vi "ODE Solver main.vi"(5 "data":variant, 7 "ODE F(X,t)":refnum<vi>, 8 "error in (no error)":errorcluster, 10 "simulation parameters":T1={"Initial Time"=0.0, "Final Time"=10.0, "Time Step"=0.1, "Absolute Tolerance"=0.001, "Relative Tolerance"=0.001, "Continuous Solver"=enum."Runge-Kutta 45 (variable)", "Discrete Time Step"=1.0, "Minimum Time Step"=1e-08, "Maximum Time Step"=1.0, "Initial Time Step"=0.01} {"Initial Time Step" min=0.0; "Maximum Time Step" min=0.0}, 11 "x0":dbl[](array[numeric])) -> (0 "error out":errorcluster, 2 "outputs":dbl[][](array[numeric]), 3 "times":dbl[](array[numeric]))   [LabVIEW 2010, in "NI_Gmath.lvlib"]
doc: "Solves ordinary differential equations with initial conditions of the following form: X'=F(X,t). You must manually select the polymorphic instance to use."
uses:
  NI_Gmath.lvlib
  SIM Diagram Parameters.ctl
  SIM Continuous Solvers.ctl
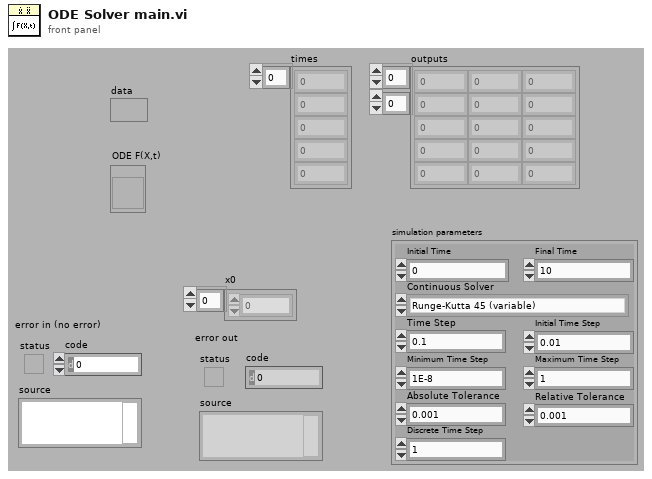
[diagram p1: front panel]
types:
  T1 = typedef "SIM Diagram Parameters.ctl" = cluster{"Initial Time":dbl, "Final Time":dbl, "Time Step":dbl, "Absolute Tolerance":dbl, "Relative Tolerance":dbl, "Continuous Solver":T2, "Discrete Time Step":dbl, "Minimum Time Step":dbl, "Maximum Time Step":dbl, "Initial Time Step":dbl}
  T2 = typedef "SIM Continuous Solvers.ctl" = enum16{"Runge-Kutta 1 (Euler)", "Runge-Kutta 2", "Runge-Kutta 3", "Runge-Kutta 4", "Runge-Kutta 23 (variable)", "Runge-Kutta 45 (variable)", "BDF (variable)", "Adams-Moulton (variable)", "Rosenbrock (variable)", "Discrete States Only"}
  T3 = typedef "SIM simulation data.ctl" = cluster{"continuous integrator":T4, "initial time":dbl, "final time":dbl, "step size":dbl, "proposed step size":dbl, "max step size":dbl, "min step size":dbl, "discrete time step":dbl, "max step ratio":dbl, "Diag Eval Stage":T5, "Substep Index":i32, "Timestep Index":dbl, "simulation time":dbl, "current timestep base":dbl, "proposed step time":dbl, "absolute tolerance":dbl, "relative tolerance":dbl, "step accepted?":bool, "step complete?":bool, "Halt?":bool, "reset integrator?":bool, "machine epsilon":dbl, "min float":dbl, "error":errorcluster, "Method Order":u32, "Finished Late [i-1]":bool, "Discrete step?":bool, "NaN and Inf check?":bool, "Final Timestep Index":dbl, "(maj+disc)or(init)?":bool, "Full Solver Reset":bool, "Execution Mode":T6, "check vector sizes?":bool, "solver handles zc?":bool, "Simulation Registry":T7, "variable step solver?":bool, "First Substep?":bool, "Continuous States?":bool}
  T4 = typedef "SIM integration method.ctl" = enum16{"RK 1 (Euler)", "Linearizer", "State Query", "Trim Eval", "Adams", "RK 3", "RK 4", "RK 45", "BDF", "RK 2", "RK 23", "Rosenbrock", "Discrete States Only"}
  T5 = typedef "SIM diagram eval stage.ctl" = enum16{"Init", "Minor Substep", "Major Substep", "Final"}
  T6 = typedef "SIMSCR Execution Mode.ctl" = u16
  T7 = typedef "SIM Simulation Registry.ctl" = cluster{"Current Idx":i32, "Node Tags":string[], "Node Headers":T8[], "Node Data":T9[], "Cont State data":T11, "DiscreteInfo":T13, "Disc State data":T14, "Registry Error":T15, "ZC Indices":i32[]}
  T8 = typedef "SIM Registry Node Header.ctl" = cluster{"Input Width":i32, "Disc ID":i32, "Num Cont St":i32, "Cont St Idx":i32, "Num Disc St":i32, "Disc St Idx":i32, "Output Width":i32}
  T9 = typedef "SIM Registry Node Record.ctl" = cluster{"Node Data":dbl[], "Node Outputs":dbl[], "Z.C. Signals":dbl[], "Z.C. Trigger Types":T10[]}
  T10 = typedef "SIM trigger type.ctl" = enum16{"rising", "falling", "either", "none"}
  T11 = typedef "SIM solver state data.ctl" = cluster{"inputs":dbl[], "outputs":dbl[], "reset":dbl[], "lower limits":dbl[], "upper limits":dbl[], "limit types":T12[], "reset types":T10[], "initial conditions":dbl[], "reset I.C.":dbl[], "limited?":bool[], "State Names":string[]}
  T12 = typedef "SIM limit type.ctl" = enum16{"upper", "lower", "both", "none"}
  T13 = typedef "SIM discrete data.ctl" = cluster{"tick period (sec)":dbl, "time (ticks)":i32, "fire?":bool[], "registry":cluster{"period (sec)":dbl[], "skew (sec)":dbl[], "period (tick)":i32[], "skew (tick)":i32[]}, "discrete \nblocks?":bool, "steps per tick":dbl, "steps to tick":dbl, "discrete \ntick?":bool}
  T14 = typedef "SIM Discrete state data.ctl" = cluster{"Disc States":dbl[], "State Names":string[]}
  T15 = typedef "SIM Simulation Registry Error.ctl" = cluster{"Error Block ID":i32, "code":i32}
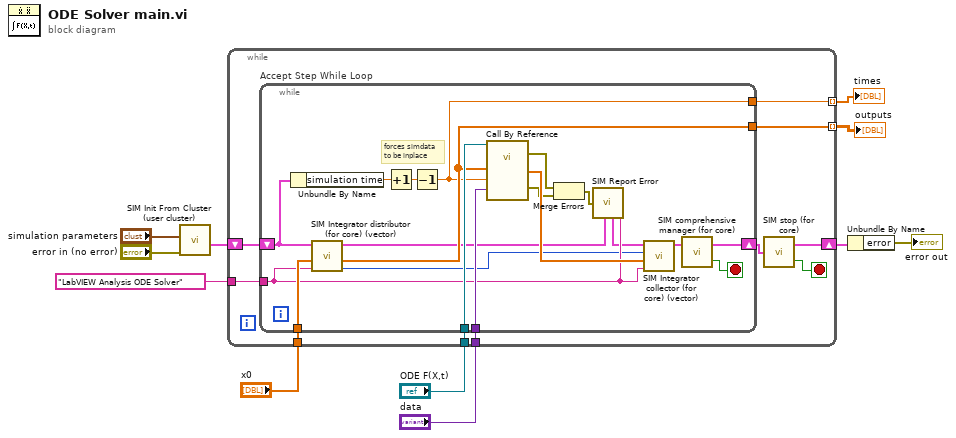
[diagram p0: block diagram]
diagram:
  n1 = call "SIM Init From Cluster (user cluster).vi"("errorin"="error in (no error)", "Sim Params"="simulation parameters") -> ("Simulation data out"=w5:T3)  [unwired: 5 in]
  n2 = while "Simulation While Loop" {
    shift-right: [w19] -> w11
    shift-left: w5 -> [w18]
    tunnel: "ODE F(X,t)" -> [w17]
    tunnel: "data" -> [w16]
    tunnel: "x0" -> [w15]
    tunnel: "LabVIEW Analysis ODE Solver" -> [w14]
    tunnel: [w13] -> w2 mode=indexing
    tunnel: [w12] -> w1 mode=indexing
    stop <- w20 stop-if-true
    n3 = while "Accept Step While Loop" {
      shift-right: [w29] -> w21
      shift-left: w18 -> [w28]
      tunnel: w17 -> [w39]
      tunnel: w16 -> [w34]
      tunnel: w15 -> [w32]
      tunnel: [w33] -> w12
      tunnel: [w25] -> w13
      tunnel: w14 -> [w31]
      stop <- w40 stop-if-true
      # "forces simdata\nto be inplace"
      n4 = Unbundle By Name(w28) -> ("simulation time"=w27:dbl)
      n5 = call "SIM Integrator distributor (for core) (vector).vi"("DNL_Simulation CallChain"=w31, "initial condition"=w32, "Simulation data"=w28) -> ("width"=w30:i32, "output"=w33:dbl[], "Simulation data out"=w22:T3)  [unwired: 6 in]
      n6 = Increment(x=w27) -> (x+1=w26:dbl)
      n7 = Decrement(x=w26) -> (x-1=w25:dbl)
      n8 = call-by-ref "?"(reference=w39, "data"=w34, "t"=w25, "x"=w33) -> (error out=w38:errorcluster, 0:"error out"=w35:errorcluster, "f'(x)"=w36:dbl[])  [unwired: 1 in, 1 out]
      n9 = Merge Errors(w38, w35) -> (w37:errorcluster)
      n10 = call "SIM Report Error.vi"("error in (no error)"=w37, "Simulation data"=w22, "DNL_Simulation CallChain"=w31) -> ("Simulation data out"=w23:T3)  [unwired: 6 in]
      n11 = call "SIM Integrator collector (for core) (vector).vi"("DNL_Simulation CallChain"=w31, "input"=w36, "width"=w30, "Simulation data"=w23) -> ("Simulation data out"=w24:T3)  [unwired: 7 in]
      n12 = call "SIM comprehensive manager (for core).vi"("Simulation data"=w24) -> ("step complete?"=w40:bool, "Simulation data out"=w29:T3)  [unwired: 1 in]
    }
    n13 = call "SIM stop (for core).vi"("Simulation data"=w21) -> ("Simulation data out"=w19:T3, "stop simulation?"=w20:bool)
  }
  "times" <- w2
  "outputs" <- w1
  n14 = Unbundle By Name(w11) -> ("error"=→"error out":errorcluster)
